vi "Create.vi"(10 "TcpPayload":T1) -> (3 "ReplyValue out":refnum<class "ReplyValue.lvclass">)   [LabVIEW 2020, in "Vecto.lvlib" / "ReplyValue.lvclass"]
uses:
  ReplyValue.lvclass
  lv-volatus/messages/TcpPayload/Data.ctl
  ReplyValue.lvclass/ReplyValue.ctl
  lv-volatus/messages/TcpPayload/TcpPayload.lvlib
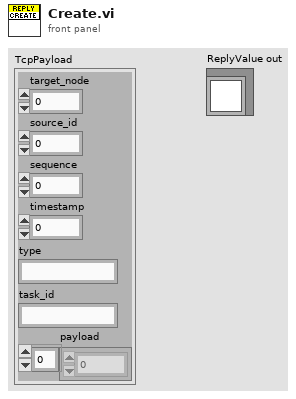
[diagram p1: front panel]
types:
  T1 = typedef "TcpPayload.lvlib/Data.ctl" = cluster{"target_node":u32, "source_id":u32, "sequence":u32, "timestamp":i64, "type":string, "task_id":string, "payload":u8[]}
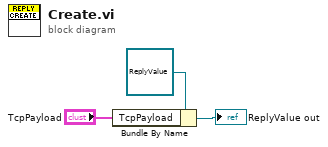
[diagram p0: block diagram]
diagram:
  n1 = Bundle By Name(cluster=refnum<class "ReplyValue.lvclass"> refnum ("ReplyValue out"), "TcpPayload"="TcpPayload") -> (→"ReplyValue out":refnum<class "ReplyValue.lvclass">)
